vi "usb capture query and req.vi"() -> (3 "function return":bool)   [LabVIEW 2018, in "Dll1_x64_191014_0.lvlib"]
doc: "__declspec(dllexport) bool usb_capture_query_and_req();"
uses:
  Dll1_x64_191014_0.lvlib
  Dll1.dll
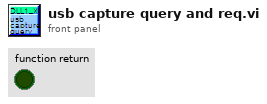
[diagram p1: front panel]
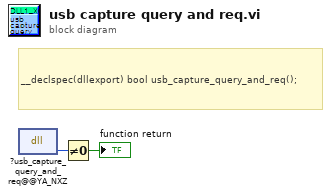
[diagram p0: block diagram]
diagram:
  # "__declspec(dllexport) bool usb_capture_query_and_req();"
  n1 = dll-call lib="PTH2zabs CUsersLenovoDesktopDHCC실험2#lux image capture_0.9.1.1_Temporaryuser.libDll1_x64_191014_0Dll1.*" fn="?usb_capture_query_and_req@@YA_NXZ"() -> (w1:u8)  [unwired: 3 in, 2 out]
  n2 = Not Equal To 0?(x=w1) -> (x != 0?=→"function return":bool)
